vi "even or odd num.vi"() -> ()   [LabVIEW 2025]
panel:
  out "odd":bool
  out "even":bool
  in  "enter a num":dbl
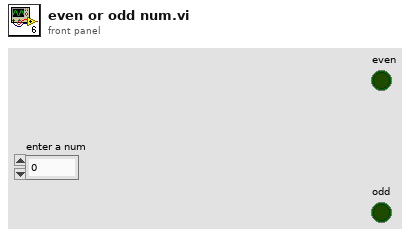
[diagram p1: front panel]
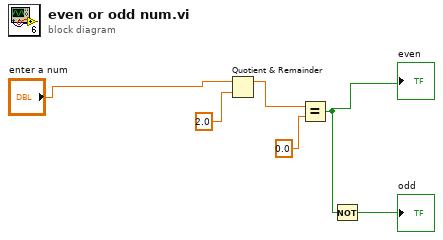
[diagram p0: block diagram]
diagram:
  n1 = Quotient & Remainder(x="enter a num", y=2.0) -> (x-y*floor(x/y)=w5:dbl)  [unwired: 1 out]
  n2 = Equal?(x=w5, y=0.0) -> (x = y?=w1:bool)
  "even" <- w1
  n3 = Not(x=w1) -> (.not. x?=→"odd":bool)
